vi "DateTime.vi"() -> (3 "date/time string":string)   [LabVIEW 2019]
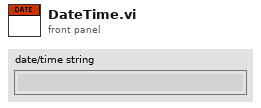
[diagram p1: front panel]
types:
  T1 = typedef "LVDateTimeRec.ctl" = cluster{"fractional second":dbl, "second":i32, "minute":i32, "hour":i32, "day of month":i32, "month":i32, "year":i32, "day of week":i32, "day of year":i32, "DST":i32}
  T2 = cluster{"fractional second":string, "second":string, "minute":string, "hour":string, "day of month":string, "month":string, "year":string, "day of week":string, "day of year":string, "DST":string}
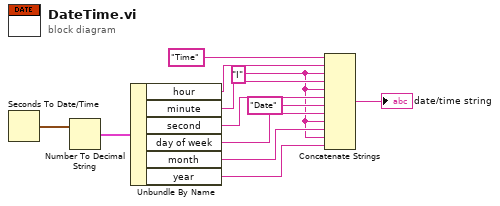
[diagram p0: block diagram]
diagram:
  w1 = "I"
  n1 = Seconds To Date/Time() -> (date time rec=w12:T1)  [unwired: 2 in]
  n2 = Number To Decimal String(number=w12) -> (decimal integer string=w11:T2)  [unwired: 1 in]
  n3 = Unbundle By Name(w11) -> ("hour"=w9:string, "minute"=w8:string, "second"=w7:string, "day of week"=w5:string, "month"=w4:string, "year"=w3:string)
  n4 = Concatenate Strings("Time", w9, w1, w8, w1, w7, "Date", w5, w1, w4, w1, w3) -> (→"date/time string":string)
